vi "TVC_Emulator.vi"() -> ()   [LabVIEW 2024]
panel:
  in  "stop":bool
  in  "TempCycleNo 2":i32
  in  "CyclesRemaining 2":i32
  in  "Period":i64=100
  in  "3A Temperature":dbl
  out "TempCycleNo":i32
  out "CyclesRemaining":i32
  out "TVC_Temperatures":waveform(dbl)[](array[waveform])
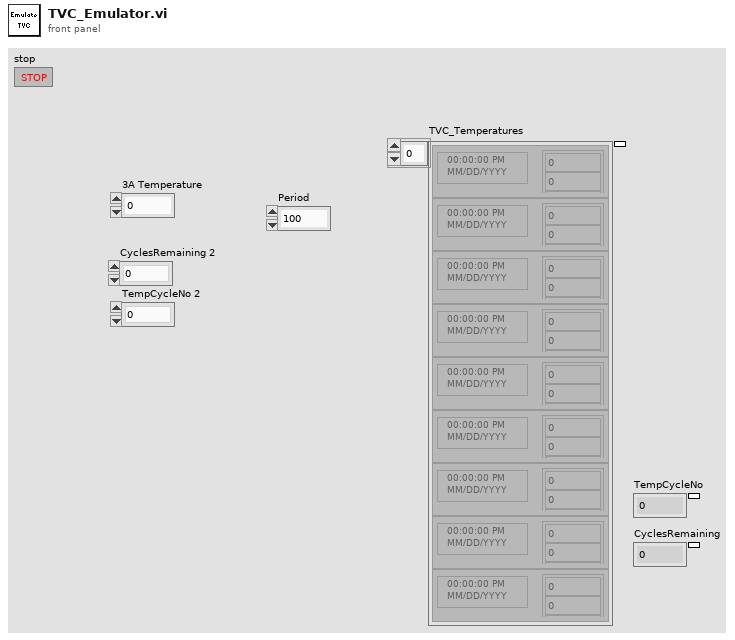
[diagram p1: front panel]
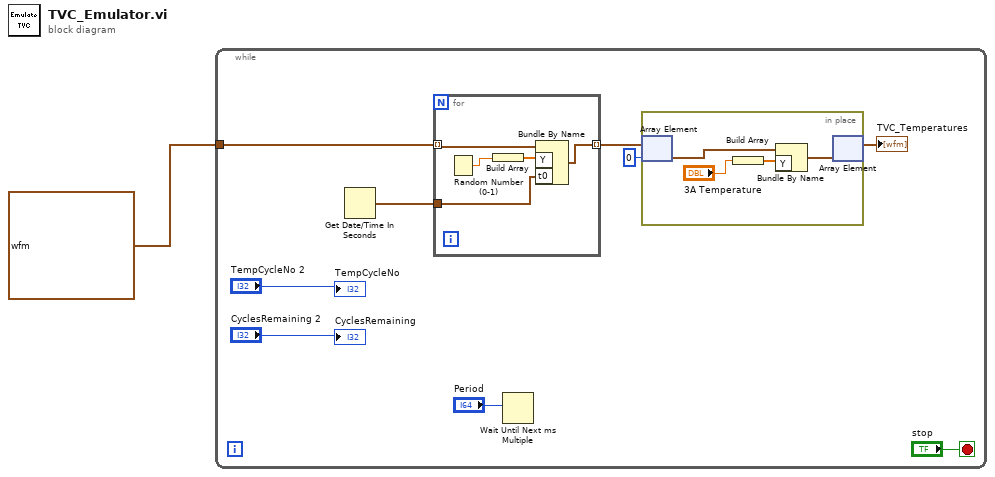
[diagram p0: block diagram]
diagram:
  n1 = while {
    tunnel: waveform(dbl)[] [{"t0"=timestamp(3819877632.797883 s since 1904-01-01), "dt"=1.0, "Y"=[-80.0], "attributes"=variant("NI_ChannelName"=variant(string "3A"))}, {"t0"=timestamp(3819877632.797883 s since 1904-01-01), "dt"=1.0, "Y"=[nan], "attributes"=variant("NI_ChannelName"=variant(string "3B"))}, {"t0"=timestamp(3819877632.797883 s since 1904-01-01), "dt"=1.0, "Y"=[-76.945], "attributes"=variant("NI_ChannelName"=variant(string "3C"))}, {"t0"=timestamp(3819877632.797883 s since 1904-01-01), "dt"=1.0, "Y"=[-75.197], "attributes"=variant("NI_ChannelName"=variant(string "3D"))}, {"t0"=timestamp(3819877632.797883 s since 1904-01-01), "dt"=1.0, "Y"=[nan], "attributes"=variant("NI_ChannelName"=variant(string "4A"))}, {"t0"=timestamp(3819877632.797883 s since 1904-01-01), "dt"=1.0, "Y"=[nan], "attributes"=variant("NI_ChannelName"=variant(string "4B"))}, {"t0"=timestamp(3819877632.797883 s since 1904-01-01), "dt"=1.0, "Y"=[-101.793], "attributes"=variant("NI_ChannelName"=variant(string "4C"))}, {"t0"=timestamp(3819877632.797883 s since 1904-01-01), "dt"=1.0, "Y"=[-72.411], "attributes"=variant("NI_ChannelName"=variant(string "4D"))}, {"t0"=timestamp(3819877632.797883 s since 1904-01-01), "dt"=1.0, "Y"=[-100.0], "attributes"=variant("NI_ChannelName"=variant(string "Target"))}] ("TVC_Temperatures 2") -> [w8]
    stop <- "stop" stop-if-true
    n2 = Get Date/Time In Seconds() -> (seconds since 1Jan1904=w6:timestamp)
    n3 = for {
      tunnel: w8 -> [w14] mode=indexing
      tunnel: [w13] -> w7 mode=indexing
      tunnel: w6 -> [w11]
      n4 = Random Number (0-1)() -> (number: 0 to 1=w12:dbl)
      n5 = Build Array(w12) -> (w15:dbl[])
      n6 = Bundle By Name(cluster=w14, "Y"=w15, "t0"=w11) -> (w13:waveform(dbl))
    }
    n7 = Wait Until Next ms Multiple(millisecond multiple="Period") -> ()  [unwired: 1 out]
    n8 = in-place {
      n9 = in-place-array #1(w7, 0) -> (w19:waveform(dbl))
      n10 = Build Array("3A Temperature") -> (w17:dbl[])
      n11 = Bundle By Name(cluster=w19, "Y"=w17) -> (w18:waveform(dbl))
      n12 = in-place-array #1(w18) -> (→"TVC_Temperatures":waveform(dbl)[])  [unwired: 1 out]
    }
    "CyclesRemaining" <- "CyclesRemaining 2"
    "TempCycleNo" <- "TempCycleNo 2"
  }
